vi "readCPC3725.vi"(8 "error in (no error)":errorcluster, 11 "connection ID":refnum<k5>) -> (0 "error out":errorcluster, 3 "value.concentration":dbl)   [LabVIEW 2017]
doc: "Use this template to build a VI to use as a subVI."
uses:
  <vilib>/regexp/Match Regular Expression.xnode
panel:
  out "whole match":string
  out "value 2":T1
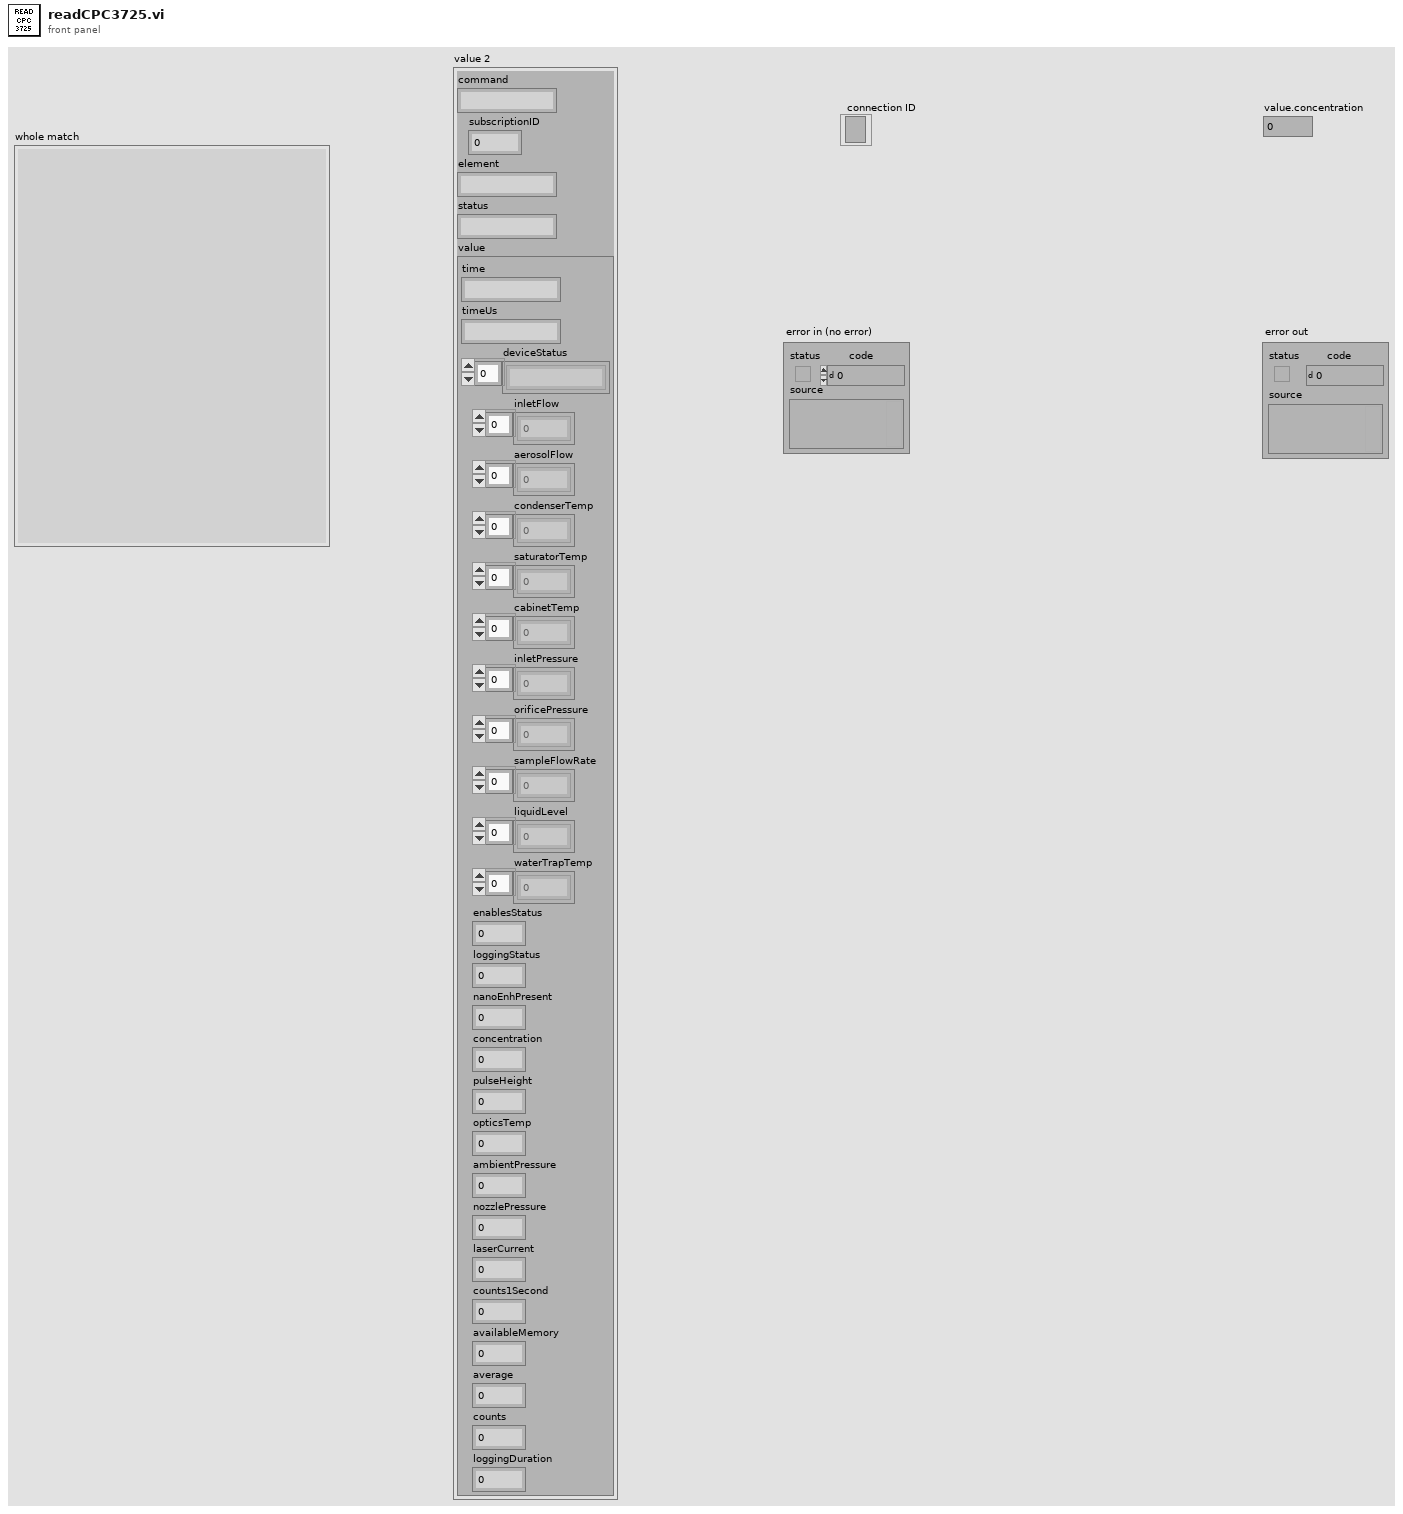
[diagram p1: front panel]
types:
  T1 = cluster{"command":string, "subscriptionID":i32, "element":string, "status":string, "value":cluster{"time":string, "timeUs":string, "deviceStatus":string[], "inletFlow":dbl[], "aerosolFlow":dbl[], "condenserTemp":dbl[], "saturatorTemp":dbl[], "cabinetTemp":dbl[], "inletPressure":dbl[], "orificePressure":dbl[], "sampleFlowRate":dbl[], "liquidLevel":dbl[], "waterTrapTemp":dbl[], "enablesStatus":i32, "loggingStatus":i32, "nanoEnhPresent":i32, "concentration":dbl, "pulseHeight":i32, "opticsTemp":dbl, "ambientPressure":dbl, "nozzlePressure":dbl, "laserCurrent":dbl, "counts1Second":dbl, "availableMemory":dbl, "average":dbl, "counts":dbl, "loggingDuration":dbl}}
  T2 = enum16{"Standard", "Buffered", "CRLF", "Immediate"}
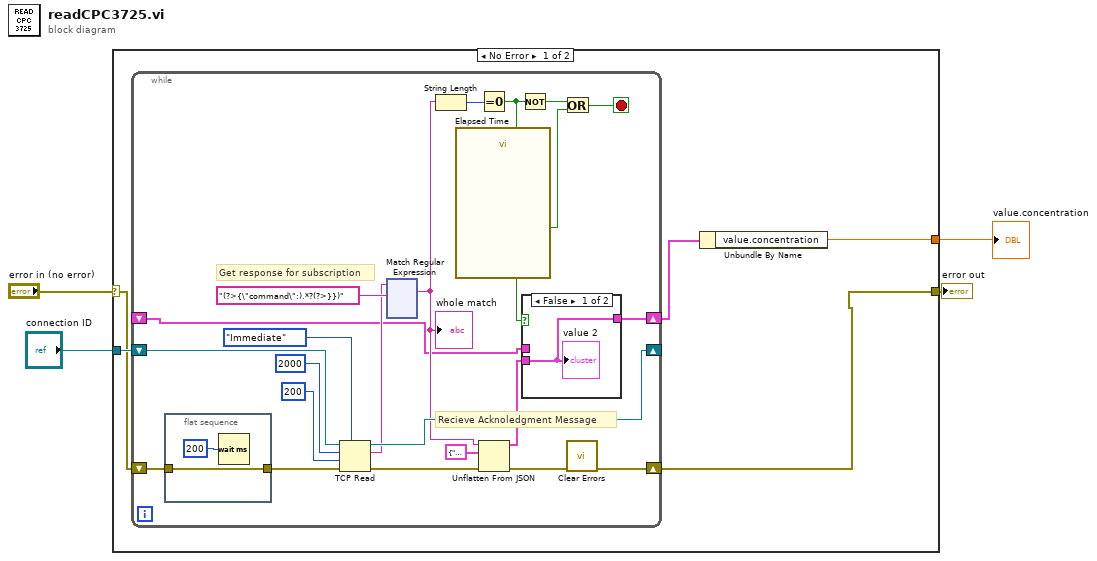
[diagram p0: block diagram]
diagram:
  n1 = case shown="No Error" "error in (no error)" {
    selector: "error in (no error)" -> [w6 w150]
    tunnel: [w7 w150] -> w3
    tunnel: "connection ID" -> [w9 _]
    tunnel: [w5 _] -> w1
    frame No Error {
      n2 = while {
        shift-right: [w27] -> _
        shift-left: w9 -> [w31]
        shift-right: [w18] -> w7
        shift-left: w6 -> [w26]
        shift-right: [w15] -> w8
        shift-left: _ -> [w14]
        stop <- w10 stop-if-true
        # "Get response for subscription"
        # "Recieve Acknoledgment Message"
        n3 = flat-sequence {
          tunnel: w26 -> [w148]
          tunnel: [w148] -> w25
          frame #0 {
            n4 = Wait (ms)(milliseconds to wait=u32 200) -> ()  [unwired: 1 out]
          }
        }
        n5 = TCP Read(connection ID=w31, bytes to read=2000, error in (no error)=w25, 7:T2."Immediate" ("mode (standard)"), 9:200 ("timeout ms (25000)")) -> (connection ID out=w27:refnum<k5>, data out=w23:string, error out=w19:errorcluster)
        n6 = xnode "Match Regular Expression"("input string"=w23, "regular expression"="(?>{\"command\":).*?(?>}})") -> ("whole match"=w17:string)  [unwired: 4 in, 4 out]
        "whole match" <- w17
        n7 = String Length(string=w17) -> (length=w16:i32)
        n8 = call "Elapsed Time"() -> ("Time has Elapsed"=w13:bool)  [unwired: 12 in, 7 out]
        n9 = Equal To 0?(x=w16) -> (x = 0?=w12:bool)
        n10 = Unflatten From JSON(JSON string=w17, type and defaults=T1 {"command"="", "subscriptionID"=0, "element"="", "status"="", "value"={"time"="", "timeUs"="", "deviceStatus"=[], "inletFlow"=[], "aerosolFlow"=[], "condenserTemp"=[], "saturatorTemp"=[], "cabinetTemp"=[], "inletPressure"=[], "orificePressure"=[], "sampleFlowRate"=[], "liquidLevel"=[], "waterTrapTemp"=[], "enablesStatus"=0, "loggingStatus"=0, "nanoEnhPresent"=0, "concentration"=0.0, "pulseHeight"=0, "opticsTemp"=0.0, "ambientPressure"=0.0, "nozzlePressure"=0.0, "laserCurrent"=0.0, "counts1Second"=0.0, "availableMemory"=0.0, "average"=0.0, "counts"=0.0, "loggingDuration"=0.0}}, error in (no error)=w19) -> (value=w21:T1, error out=w20:errorcluster)  [unwired: 4 in]
        n11 = Not(x=w12) -> (.not. x?=w11:bool)
        n12 = case shown="False" w12 {
          tunnel: w21 -> [w32 _]
          tunnel: [w32 w33] -> w15
          tunnel: w14 -> [_ w33]
          frame False {
            "value 2" <- w32
          }
          frame True {
          }
        }
        n13 = Or(x=w11, y=w13) -> (x .or. y?=w10:bool)
        n14 = call <vilib>:"Clear Errors.vi"("error in (no error)"=w20) -> ("error out"=w18:errorcluster)  [unwired: 5 in, 1 out]
      }
      n15 = Unbundle By Name(w8) -> ("value.concentration"=w5:dbl)
    }
    frame Error {
    }
  }
  "error out" <- w3
  "value.concentration" <- w1
